vi "Apply VacuumLine Config Obj by Label.vi"(8 "error in (no error)":errorcluster, 10 "VacuumLine Configuration Obj":refnum<class "VacuumLine Configuration.lvclass">, 11 "VacuumLines Configuration in":refnum<class "VacuumLines Configuration.lvclass">) -> (0 "error out":errorcluster, 3 "VacuumLines Configuration out":refnum<class "VacuumLines Configuration.lvclass">)   [LabVIEW 2016, in "Hardware.lvlib" / "VacuumLine.lvlib" / "VacuumLines Configuration.lvclass"]
uses:
  <userlib>/Common Components/Hardware/Abstract System/VacuumLine/VacuumLines Configuration/VacuumLines Configuration.lvclass
  <userlib>/Common Components/Hardware/Abstract System/VacuumLine/VacuumLine Config/VacuumLine Configuration.lvclass
  <userlib>/Common Components/Hardware/Abstract System/VacuumLine/VacuumLines Configuration/VacuumLines Configuration.lvclass/VacuumLines Configuration.ctl
  <userlib>/Common Components/Hardware/Abstract System/VacuumLine/VacuumLine Config/VacuumLine Configuration.lvclass/VacuumLine Configuration.ctl
  <userlib>/Common Components/Hardware/Abstract System/VacuumLine/VacuumLines/VacuumLines.lvclass/VacuumLines.ctl
  <userlib>/Common Components/Hardware/Abstract System/VacuumLine/VacuumLine/VacuumLine.lvclass/VacuumLine.ctl
  <userlib>/Common Components/Hardware/Abstract System/VacuumLine/VacuumLine/VacuumLine.lvclass
  <userlib>/Common Components/Hardware/Abstract System/VacuumLine/VacuumLines/VacuumLines.lvclass
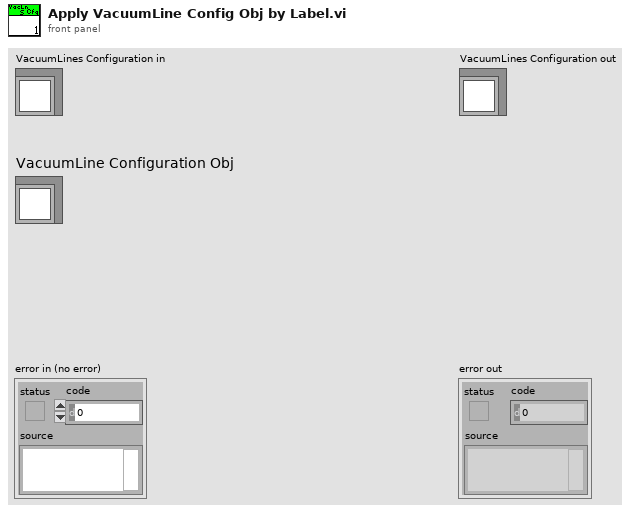
[diagram p1: front panel]
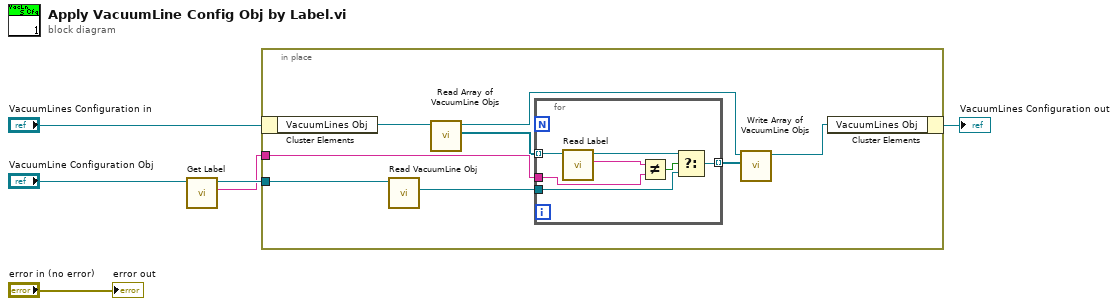
[diagram p0: block diagram]
diagram:
  n1 = call <userlib>:"Get Label.vi"("VacuumLine Configuration in"="VacuumLine Configuration Obj") -> ("Label"=w1:string, "VacuumLine Configuration out"=w2:refnum<class "VacuumLine Configuration.lvclass">)  [unwired: 8 in, 1 out]
  n2 = in-place {
    in-place-border: w1 -> [w14]
    in-place-border: w2 -> [w13]
    n3 = in-place-cluster #1("VacuumLines Configuration in") -> ("VacuumLines Obj"=w12:refnum<class "VacuumLines.lvclass">)
    n4 = call <userlib>:"Read VacuumLine Obj.vi"("VacuumLine Configuration in"=w13) -> ("Hardware.lvlib:VacuumLine.lvlib:VacuumLine.lvclass"=w9:refnum<class "VacuumLine.lvclass">)  [unwired: 8 in, 2 out]
    n5 = call <userlib>:"Read Array of VacuumLine Objs.vi"("VacuumLines in"=w12) -> ("Array of VacuumLine Objs"=w10:refnum<class "VacuumLine.lvclass">[], "VacuumLines out"=w7:refnum<class "VacuumLines.lvclass">)  [unwired: 9 in]
    n6 = for {
      tunnel: w10 -> [w21] mode=indexing
      tunnel: w14 -> [w20]
      tunnel: w9 -> [w17]
      tunnel: [w16] -> w11 mode=indexing
      n7 = call <userlib>:"Read Label.vi"("VacuumLine in"=w21) -> ("Label"=w15:string, "VacuumLine out"=w18:refnum<class "VacuumLine.lvclass">)  [unwired: 8 in, 1 out]
      n8 = Not Equal?(x=w15, y=w20) -> (x != y?=w19:bool)
      n9 = Select(t=w18, s=w19, f=w17) -> (s? t:f=w16:refnum<class "VacuumLine.lvclass">)
    }
    n10 = call <userlib>:"Write Array of VacuumLine Objs.vi"("Array of VacuumLine Objs"=w11, "VacuumLines in"=w7) -> ("VacuumLines out"=w8:refnum<class "VacuumLines.lvclass">)  [unwired: 9 in]
    n11 = in-place-cluster #1("VacuumLines Obj"=w8) -> (→"VacuumLines Configuration out":refnum<class "VacuumLines Configuration.lvclass">)
  }
  "error out" <- "error in (no error)"
